vi "Program Path to string.vi"(8 "error in":errorcluster, 11 "MPLab in":refnum<class "MPLab.lvclass">) -> (0 "error out":errorcluster, 3 "MPLab out":refnum<class "MPLab.lvclass">)   [LabVIEW 2018, in "MPLab.lvlib" / "MPLab.lvclass"]
uses:
  MPLab.lvclass
  MPLab.lvclass/MPLab.ctl
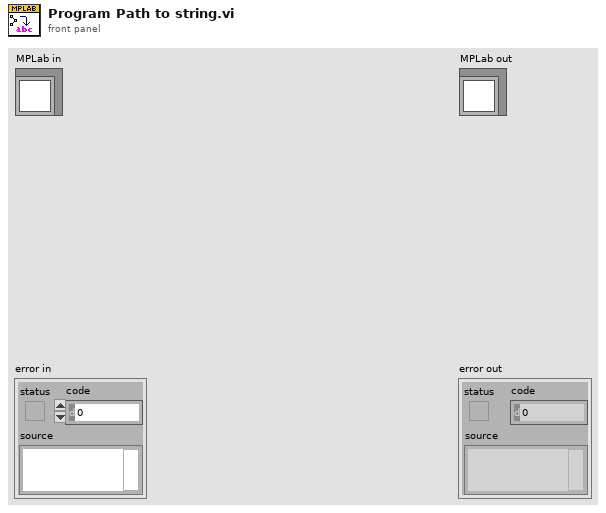
[diagram p1: front panel]
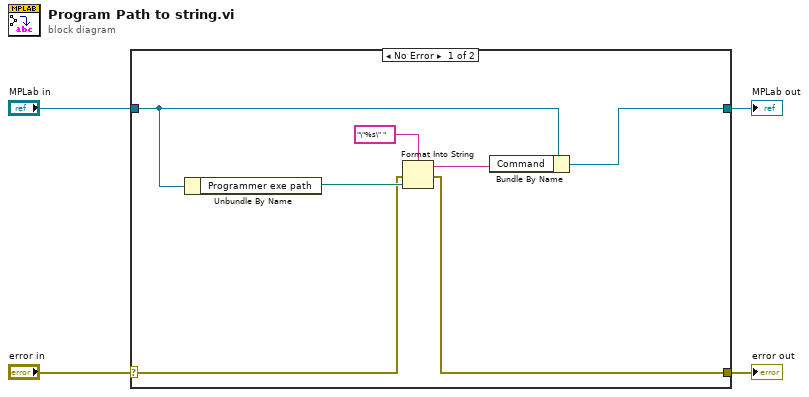
[diagram p0: block diagram]
diagram:
  n1 = case shown="No Error" "error in" {
    selector: "error in" -> [w6 w13]
    tunnel: [w5 w13] -> w3
    tunnel: [w8 w12] -> w1
    tunnel: "MPLab in" -> [w9 w12]
    frame No Error {
      n2 = Unbundle By Name(w9) -> ("Programmer exe path"=w11:path)
      n3 = Format Into String(format string="\"%s\" ", error in=w6, w11) -> (resulting string=w7:string, error out=w5:errorcluster)  [unwired: 1 in]
      n4 = Bundle By Name(cluster=w9, "Command"=w7) -> (w8:refnum<class "MPLab.lvclass">)
    }
    frame Error {
    }
  }
  "error out" <- w3
  "MPLab out" <- w1
